vi "Test resample.vi"() -> ()   [LabVIEW 2016]
uses:
  LabActor/Post-Processors/Line Detector/Line Detector Configuration.ctl
panel:
  in  "Frequency scale":dbl=1000.0
  out "XY Graph":T1(graph)
  in  "File":path=path "C:/Data/April_2017/042017/ru112_042017.tdms"
  in  "Line Detector Configuration":T2={"Peak width guess"=500.0, "Background removal"=enum."High-pass", "Smoothing"=enum."Low-pass", "Smooth window"=200.0, "Relative threshold"=0.2, "Finder algorithm"=enum."Wavelet", "Bgd window"=50000.0, "Spectrum recorder module name"="Spectrum Recorder", "Fit window"=1000.0, "Initial fit guess"=enum."Peak finder", "...with header "="", "Follow\npeaks"=FALSE, "Re-sample"=nan, "rusin\n.dat"=enum."NONE"} {"Re-sample" format="%#_6pHz"; "Fit window" format="%#_6pHz"; "Bgd window" format="%#_6pHz"; "Smooth window" format="%#_6pHz"; "Peak width guess" format="%#_6pHz"}
  # "Peak finder config"
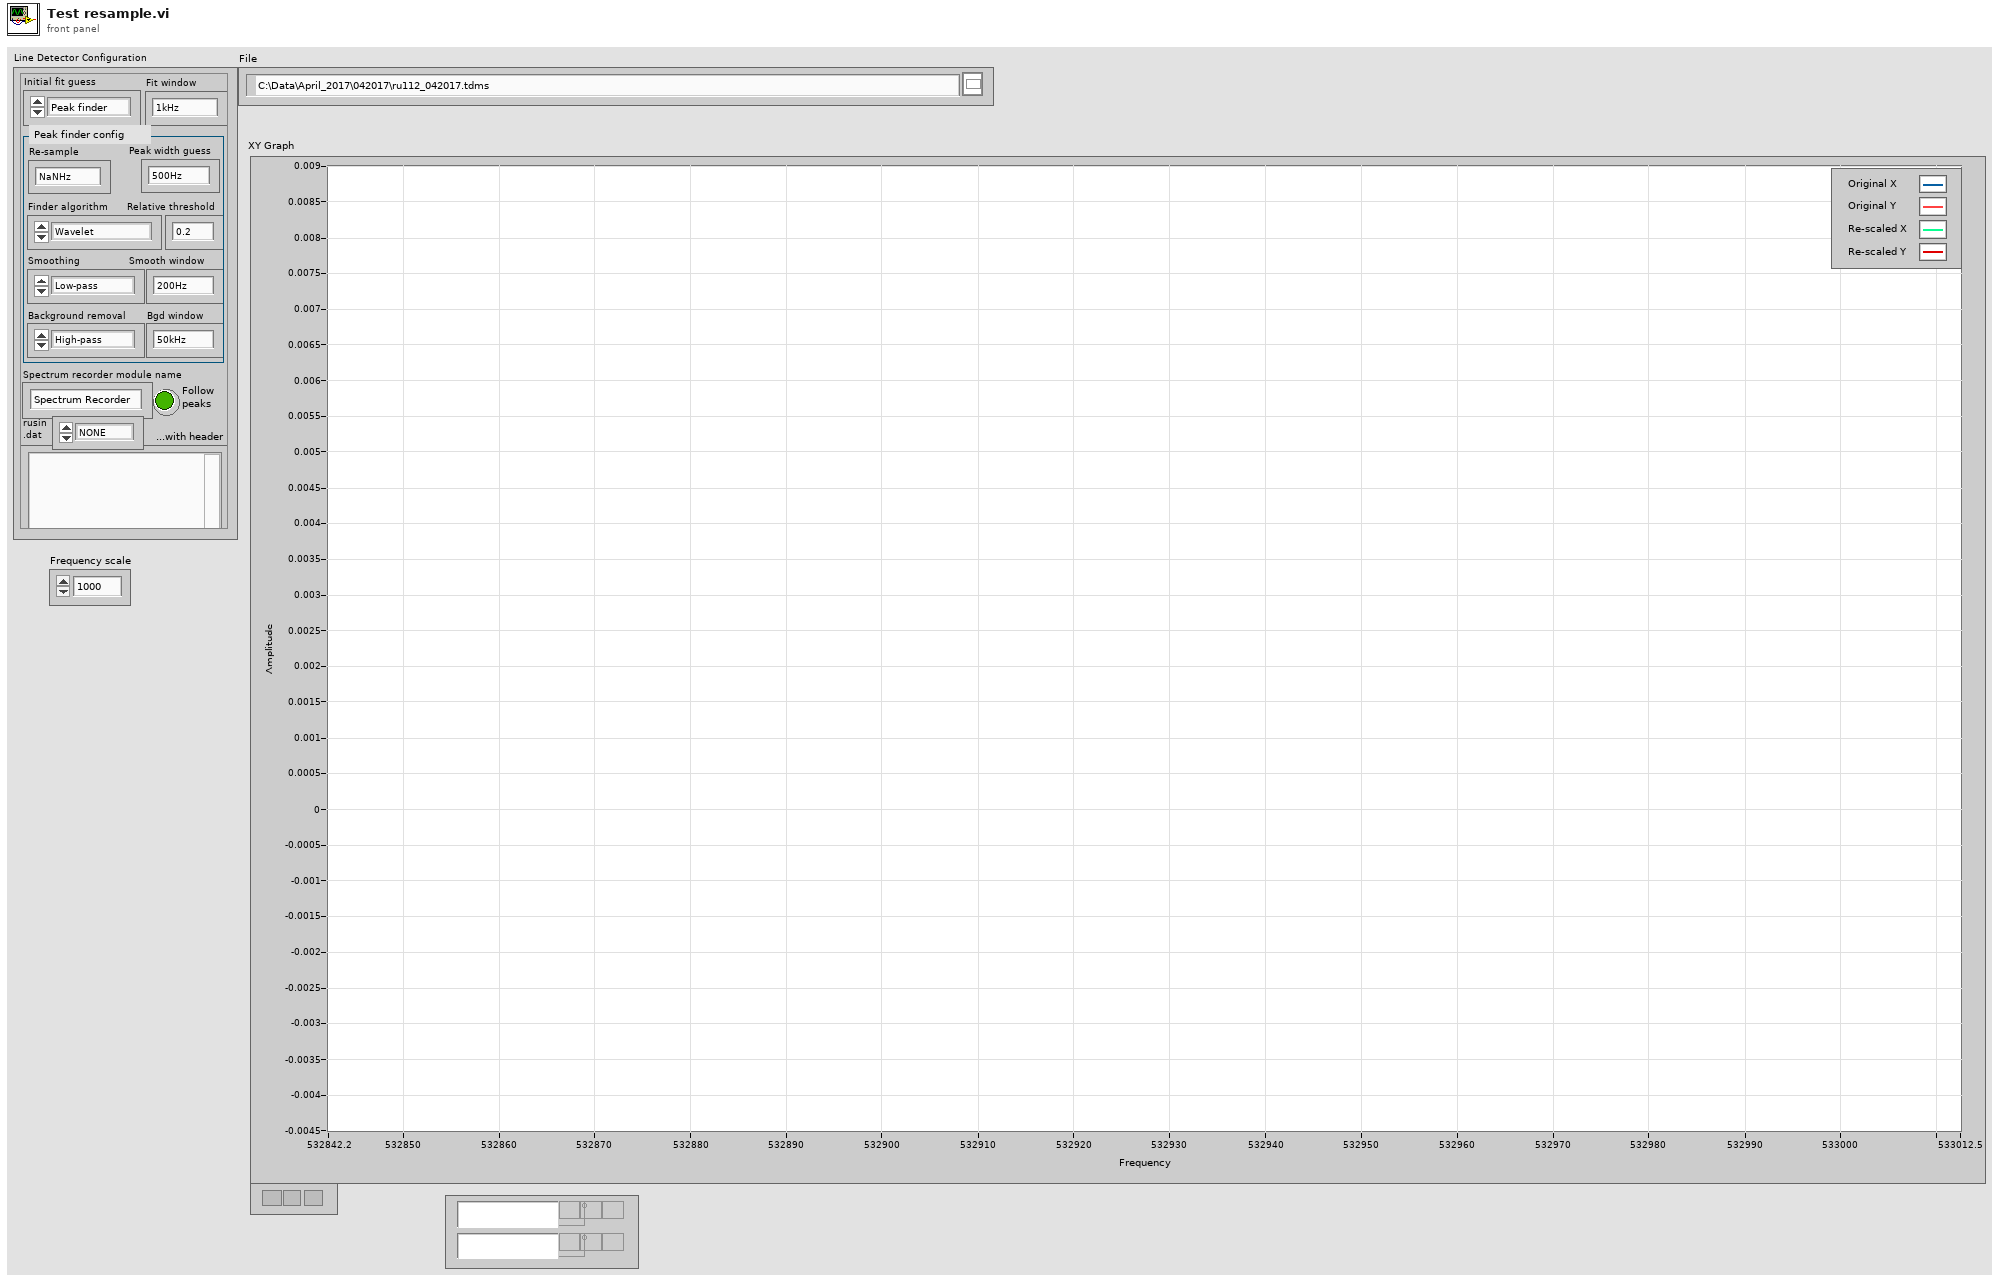
[diagram p1: front panel]
types:
  T1 = cluster{"Frequency out":dbl[], "Signal Y out":dbl[]}[]
  T2 = typedef "Line Detector Configuration.ctl" = cluster{"Peak width guess":dbl, "Background removal":enum16{"NONE", "High-pass", "Detrend"}, "Smoothing":enum16{"NONE", "Low-pass", "Denoise"}, "Smooth window":dbl, "Relative threshold":dbl, "Finder algorithm":enum16{"Basic", "Wavelet", "Wavelet+detrend"}, "Bgd window":dbl, "Spectrum recorder module name":string, "Fit window":dbl, "Initial fit guess":enum16{"Peak finder", "Last fit"}, "...with header ":string, "Follow\npeaks":bool, "Re-sample":dbl, "rusin\n.dat":enum16{"NONE", "DINES/cm2", "GPa"}}
  T3 = cluster{"Frequency out":dbl[], "Signal X out":dbl[]}
  T4 = cluster{"Frequency out":dbl[], "Signal Y out":dbl[]}
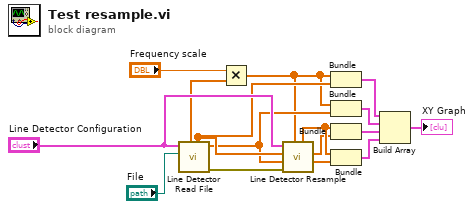
[diagram p0: block diagram]
diagram:
  n1 = call "Line Detector Read File.vi"("File"="File", "Line Detector Configuration"="Line Detector Configuration") -> ("error out"=w14:errorcluster, "Signal Y"=w6:dbl[], "Signal X"=w7:dbl[], "Frequency"=w9:dbl[])  [unwired: 2 in, 4 out]
  n2 = Multiply(x="Frequency scale", y=w9) -> (x*y=w2:dbl[])
  n3 = call "Line Detector Resample.vi"("Frequency"=w2, "error in (no error)"=w14, "Signal Y"=w6, "Signal X"=w7, "Line Detector Configuration"="Line Detector Configuration") -> ("Signal Y out"=w4:dbl[], "Signal X out"=w5:dbl[], "Frequency out"=w8:dbl[])  [unwired: 3 in, 1 out]
  n4 = Bundle(w2, "Signal X"=w7) -> (w13:cluster{dbl[], "Signal X":dbl[]})  [unwired: 1 in]
  n5 = Bundle(w2, "Signal Y"=w6) -> (w12:cluster{dbl[], "Signal Y":dbl[]})  [unwired: 1 in]
  n6 = Bundle("Frequency out"=w8, "Signal X out"=w5) -> (w11:T3)  [unwired: 1 in]
  n7 = Bundle("Frequency out"=w8, "Signal Y out"=w4) -> (w10:T4)  [unwired: 1 in]
  n8 = Build Array(w13, w12, w11, w10) -> (→"XY Graph":T1)
